vi "Test Ag87xx.vi"() -> ()   [LabVIEW 2020, in "VNA-Ag87xx.lvclass"]
uses:
  VNA-Ag87xx.lvclass
  Controls/Sparameter cluster.ctl
  C:/Sandbox/RF Bench/Source Code/WiSpry Test Framework/Instruments/Instrument.lvclass
  Instrument.lvclass/Instrument.ctl
  Instrument.lvclass
  Vector Network Analyzer.lvclass
panel:
  out "S parameters":T1[](array[typedef])
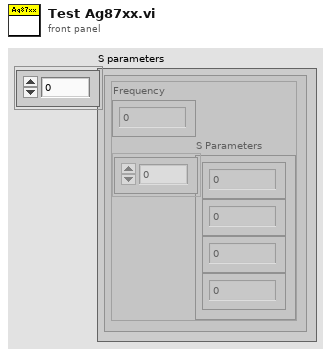
[diagram p1: front panel]
types:
  T1 = typedef "Vector Network Analyzer.lvclass/Sparameter cluster.ctl" = cluster{"Frequency":dbl, "S Parameters":cdb[]}
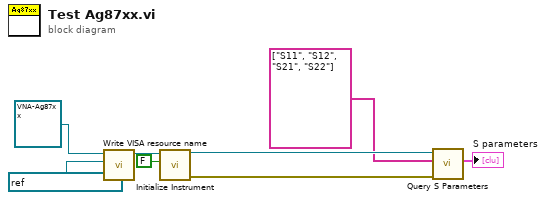
[diagram p0: block diagram]
diagram:
  n1 = call "Write VISA resource name.vi"("VISA resource name"=refnum<visa-resource-name> "GPIB0::10::INSTR", "Instrument in"=refnum<class "VNA-Ag87xx.lvclass"> refnum ("VNA-Ag87xx.lvclass")) -> ("Instrument out"=w7:refnum<class "VNA-Ag87xx.lvclass">)  [unwired: 9 in]
  n2 = call-dynamic "Initialize Instrument.vi"("Reset"=FALSE, "VNA-Ag87xx in"=w7) -> ("error out"=w3:errorcluster, "VNA-Ag87xx out"=w4:refnum<class "VNA-Ag87xx.lvclass">)  [unwired: 8 in]
  n3 = call-dynamic "Query S Parameters.vi"("error in (no error)"=w3, "Sparameters (string)"=string[] ["S11", "S12", "S21", "S22"], "VNA-Ag87xx in"=w4) -> ("S parameters"=→"S parameters":T1[])  [unwired: 6 in, 2 out]
